vi "读取数值.vi"(8 "error in (no error)":errorcluster, 10 "Slave ID":u8=1, 11 "MB session in":refnum<class "MB_Master.lvclass">) -> (0 "error out":errorcluster, 2 "读取值":T1, 3 "MB session out":refnum<class "MB_Master.lvclass">)   [LabVIEW 2016, in "流量计集成.lvlib" / "LSS-100X流量计.lvlib"]
uses:
  <vilib>/Plasmionique/MB Master/MB_Master/MB_Master.lvclass
  <vilib>/Plasmionique/MB Master/MB Master.lvlib
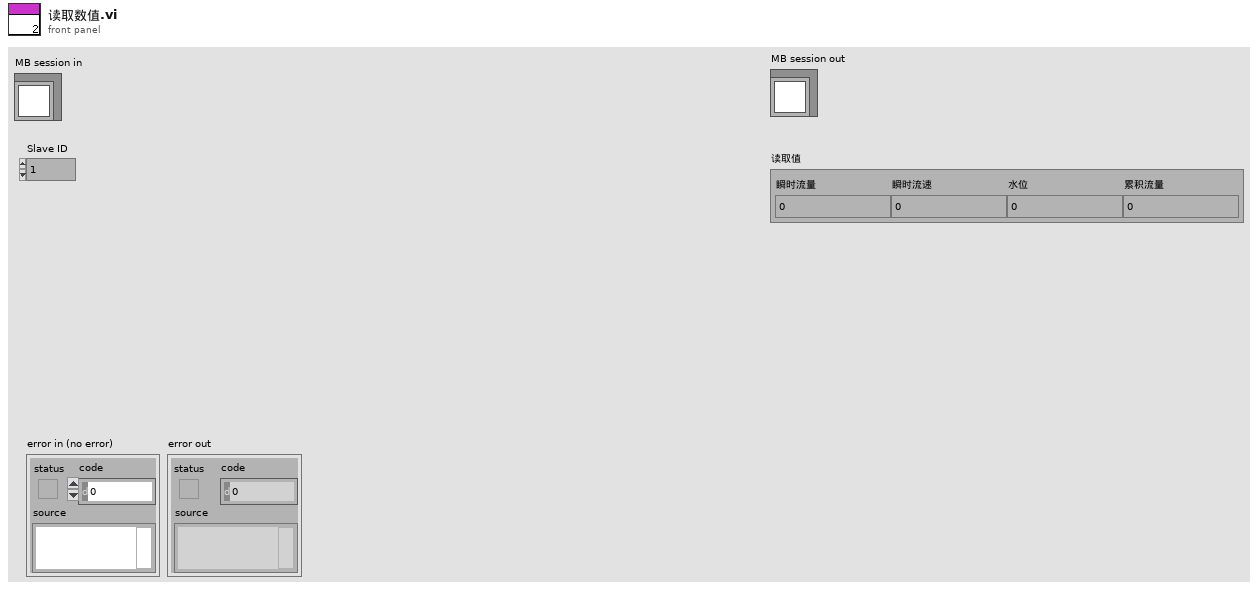
[diagram p1: front panel]
types:
  T1 = typedef "流量计集成.lvlib/LSS-100X流量计.lvlib/读取值.ctl" = cluster{"瞬时流量":sgl, "瞬时流速":sgl, "水位":sgl, "累积流量":i32}
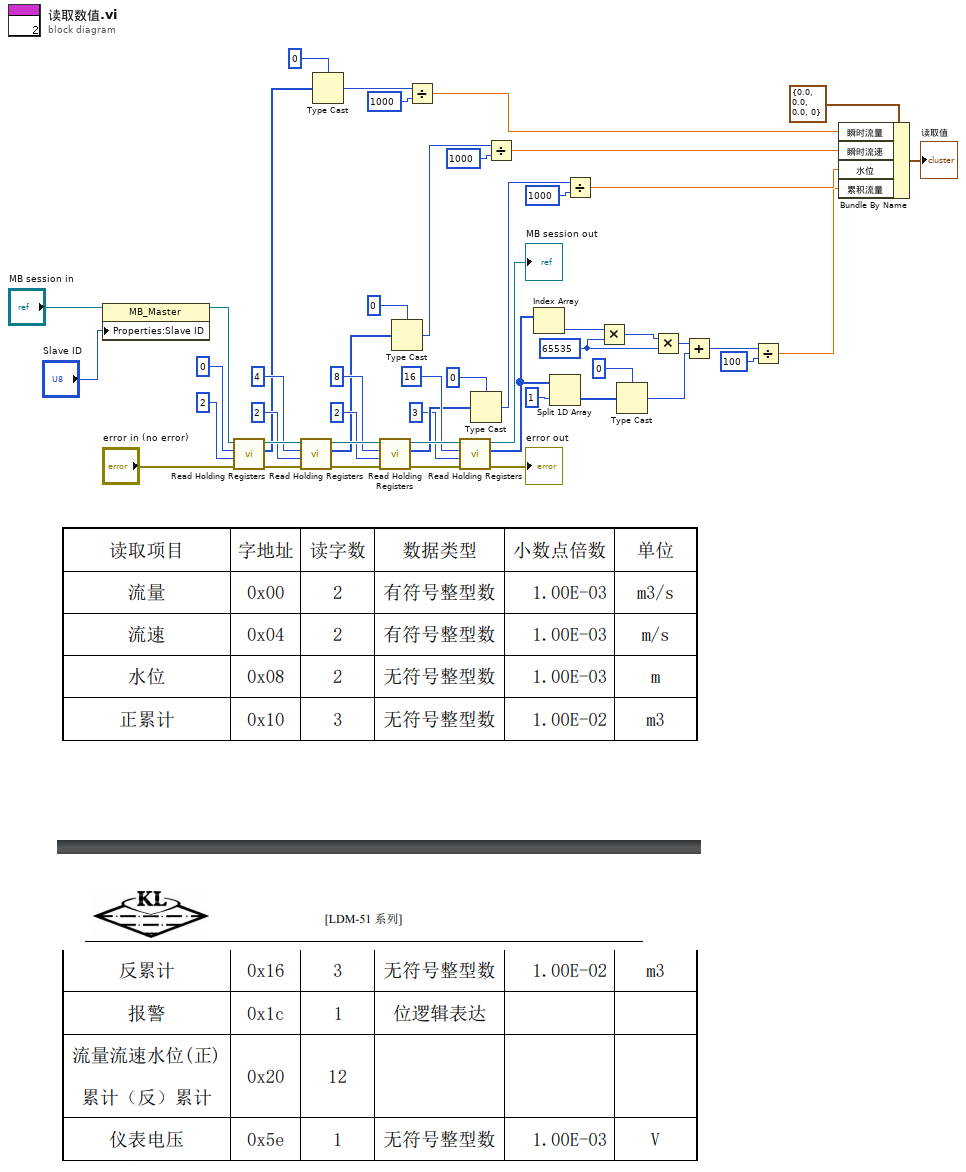
[diagram p0: block diagram]
diagram:
  w15 = u32 65535 ("y")
  n1 = property class="MB_Master"(reference="MB session in", "Properties:Slave ID"="Slave ID") -> (reference out=w26:refnum<class "MB_Master.lvclass">)  [unwired: 1 in, 1 out]
  n2 = call <vilib>:"Read Holding Registers.vi"("error in (no error)"="error in (no error)", "quantity"=u16 2, "starting address"=u16 0, "MB session in"=w26) -> ("error out"=w46:errorcluster, "Registers"=w36:u16[], "MB session out"=w47:refnum<class "MB_Master.lvclass">)  [unwired: 5 in]
  n3 = call <vilib>:"Read Holding Registers.vi"("error in (no error)"=w46, "quantity"=u16 2, "starting address"=u16 4, "MB session in"=w47) -> ("error out"=w40:errorcluster, "Registers"=w35:u16[], "MB session out"=w43:refnum<class "MB_Master.lvclass">)  [unwired: 5 in]
  n4 = Type Cast(type=0, x=w36) -> (*(type *) &x=w25:i32)
  n5 = call <vilib>:"Read Holding Registers.vi"("error in (no error)"=w40, "quantity"=u16 2, "starting address"=u16 8, "MB session in"=w43) -> ("error out"=w38:errorcluster, "Registers"=w33:u16[], "MB session out"=w39:refnum<class "MB_Master.lvclass">)  [unwired: 5 in]
  n6 = Type Cast(type=0, x=w35) -> (*(type *) &x=w23:i32)
  n7 = Divide(x=w25, y=1000) -> (x/y=w4:dbl)
  n8 = call <vilib>:"Read Holding Registers.vi"("error in (no error)"=w38, "quantity"=u16 3, "starting address"=u16 16, "MB session in"=w39) -> ("error out"=→"error out":errorcluster, "Registers"=w22:u16[], "MB session out"=→"MB session out":refnum<class "MB_Master.lvclass">)  [unwired: 5 in]
  n9 = Type Cast(type=0, x=w33) -> (*(type *) &x=w24:i32)
  n10 = Divide(x=w23, y=1000) -> (x/y=w3:dbl)
  n11 = Index Array(array=w22) -> (element=w17:u16)  [unwired: 1 in]
  n12 = Split 1D Array(array=w22, index=1 ("索引")) -> (second subarray=w20:u16[])  [unwired: 1 out]
  n13 = Divide(x=w24, y=1000) -> (x/y=w2:dbl)
  n14 = Multiply(x=w17, y=w15) -> (x*y=w16:u32)
  n15 = Type Cast(type=0, x=w20) -> (*(type *) &x=w18:i32)
  n16 = Multiply(x=w16, y=w15) -> (x*y=w14:u32)
  n17 = Add(x=w14, y=w18) -> (x+y=w13:u32)
  n18 = Divide(x=w13, y=100) -> (x/y=w1:dbl)
  n19 = Bundle By Name(cluster=T1 {"瞬时流量"=0.0, "瞬时流速"=0.0, "水位"=0.0, "累积流量"=0} ("读取值"), "瞬时流量"=w4, "瞬时流速"=w3, "水位"=w2, "累积流量"=w1) -> (→"读取值":T1)
